vi "Create Table Data.vi"(8 "error in (no error)":errorcluster, 10 "Table Control":refnum<vi>, 11 "Results":T1(array[cluster])) -> (0 "error out":errorcluster, 3 "Results out":T1(array[cluster]))   [LabVIEW 2025, in "Geocoding Actor.lvlib" / "Geocoding.lvclass"]
uses:
  UI/UI/UI.lvclass/UI.ctl
  Geocoding.lvclass
  Geocoding.lvclass/Geocoding.ctl
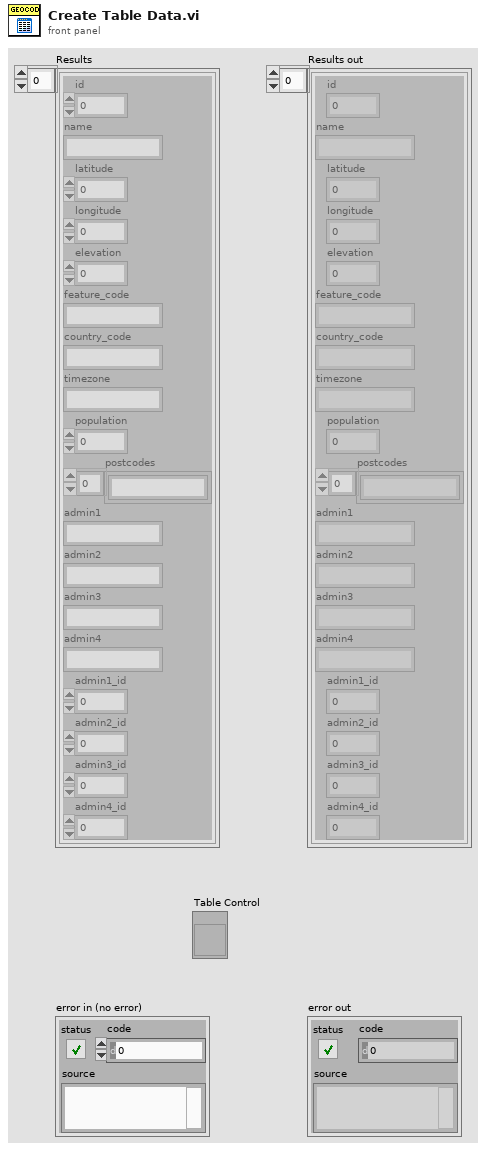
[diagram p1: front panel]
types:
  T1 = cluster{"id":i32, "name":string, "latitude":dbl, "longitude":dbl, "elevation":dbl, "feature_code":string, "country_code":string, "timezone":string, "population":i32, "postcodes":string[], "admin1":string, "admin2":string, "admin3":string, "admin4":string, "admin1_id":i32, "admin2_id":i32, "admin3_id":i32, "admin4_id":i32}[]
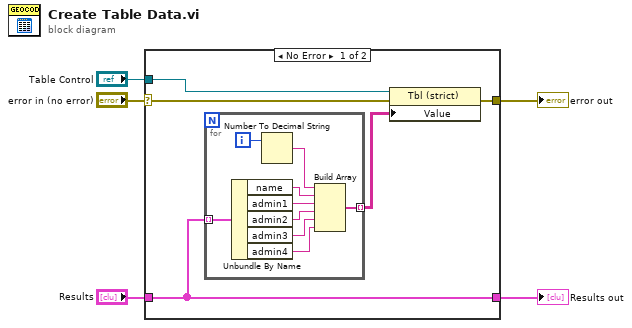
[diagram p0: block diagram]
diagram:
  n1 = case shown="No Error" "error in (no error)" {
    selector: "error in (no error)" -> [w8 w21]
    tunnel: "Results" -> [w6 w20]
    tunnel: "Table Control" -> [w10 _]
    tunnel: [w7 w21] -> w3
    tunnel: [w6 w20] -> w2
    frame No Error {
      n2 = for {
        tunnel: w6 -> [w19] mode=indexing
        tunnel: [w11] -> w9 mode=indexing
        i -> [w18]
        n3 = Unbundle By Name(w19) -> ("name"=w17:string, "admin1"=w16:string, "admin2"=w14:string, "admin3"=w13:string, "admin4"=w12:string)
        n4 = Number To Decimal String(number=w18) -> (decimal integer string=w15:string)  [unwired: 1 in]
        n5 = Build Array(w15, w17, w16, w14, w13, w12) -> (w11:string[])
      }
      n6 = property class="Tbl (strict)"(reference=w10, error in=w8, "Value"=w9) -> (error out=w7:errorcluster)  [unwired: 1 out]
    }
    frame Error {
    }
  }
  "Results out" <- w2
  "error out" <- w3
